vi "Teleop.vi"(10 "Match Info":T1={"Autonomous Elapsed Seconds"=0.0, "TeleOp Elapsed Seconds"=0.0, "Disabled Elapsed Seconds"=0.0, "Visited Autonomous"=FALSE, "Visited TeleOp"=FALSE, "Visited Disabled"=FALSE, "Autonomous Settings"={"Autonomous Style"=enum."Independent", "VI Refnum"=refnum}}, 11 "Call Context":T2) -> ()   [LabVIEW 2016]
doc: "This VI is called for each TeleOp packet received from the DS where the robot is not disabled. It is often used to read from the joysticks and update I/O or to update setpoints for timed control loops. It should complete and return within 20 milliseconds or it may miss DS packets."
uses:
  <vilib>/Rock Robotics/WPI/DriverStation/WPI_DriverStationDerivedRobotMode.ctl
  <vilib>/Rock Robotics/WPI/DriverStation/WPI_DriverStationMatch Info.ctl
  <vilib>/Rock Robotics/WPI/Solenoid/WPI_SolenoidValue.ctl
  <vilib>/Rock Robotics/WPI/Relay/WPI_RelayValue.ctl
  <vilib>/Rock Robotics/Network Tables/NT Read Boolean.vi
  <vilib>/Rock Robotics/Network Tables/NT Read Number.vi
  <vilib>/Rock Robotics/WPI/Utilities/WPI_GetSetVariantRefNum.vi
  <vilib>/Rock Robotics/Network Tables/NT Write Boolean Array.vi
  <vilib>/Rock Robotics/Network Tables/NT Write Numeric Array.vi
  <vilib>/Rock Robotics/WPI/RobotDrive/WPI_RobotDriveMecanumDrive_Cartesian.vi
  <vilib>/Rock Robotics/Network Tables/NT Write Boolean.vi
  <vilib>/Rock Robotics/WPI/Solenoid/WPI_SolenoidSetEnum.vi
  <vilib>/Rock Robotics/Network Tables/NT Write Number.vi
panel:
  out "Sample Slider 0":dbl(slide) scale=0.0..5.0
  out "Sample Boolean 1":bool
  out "Sample Boolean 0":bool
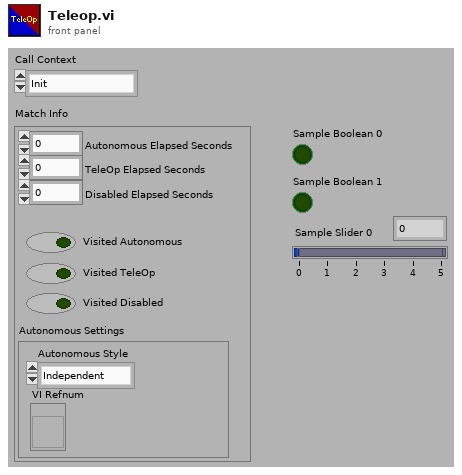
[diagram p1: front panel]
types:
  T1 = typedef "WPI_DriverStationMatch Info.ctl" = cluster{"Autonomous Elapsed Seconds":dbl, "TeleOp Elapsed Seconds":dbl, "Disabled Elapsed Seconds":dbl, "Visited Autonomous":bool, "Visited TeleOp":bool, "Visited Disabled":bool, "Autonomous Settings":cluster{"Autonomous Style":enum16{"Iterative", "Independent"}, "VI Refnum":refnum<vi>}}
  T2 = typedef "WPI_DriverStationDerivedRobotMode.ctl" = enum16{"Init", "Execute", "Stop"}
  T3 = typedef "WPI_SolenoidValue.ctl" = enum16{"Off", "On", "Forward", "Reverse"}
  T4 = typedef "WPI_MotorControlDeviceRef.ctl" = cluster{"DeviceStatus":errorcluster, "Type":T5, "PWM":cluster{"PWM Channel":T6, "DeadBand":T7}, "CAN":cluster{"Device Number":u8, "SetOutput VI Ref":variant, "GetOutput VI Ref":variant, "Enable VI Ref":variant, "Disable VI Ref":variant, "Data":variant}, "Invert":bool}
  T5 = typedef "WPI_MotorControlType.ctl" = enum16{"PWM", "CAN"}
  T6 = typedef "FPGA_DIOPWMChannel.ctl" = enum8{"PWM 0", "PWM 1", "PWM 2", "PWM 3", "PWM 4", "PWM 5", "PWM 6", "PWM 7", "PWM 8", "PWM 9", "PWM MXP 0", "PWM MXP 1", "PWM MXP 2", "PWM MXP 3", "PWM MXP 4", "PWM MXP 5", "PWM MXP 6", "PWM MXP 7", "PWM MXP 8", "PWM MXP 9", "Invalid"}
  T7 = typedef "WPI_PWMDeadband.ctl" = cluster{"Name":string, "maxPositivePwm":i32, "minPositivePwm":i32, "centerPwm":i32, "maxNegativePwm":i32, "minNegativePwm":i32, "angularRange":u16}
  T8 = typedef "WPI_JoystickDevRef.ctl" = cluster{"Device":T9}
  T9 = typedef "WPI_JoystickDeviceEnum.ctl" = enum16{"USB 0", "USB 1", "USB 2", "USB 3", "USB 4", "USB 5"}
  T10 = typedef "WPI_SolenoidDevRef.ctl" = cluster{"DevStatus":errorcluster, "Pneumatics Control Module":u8, "Forward Solenoid Channel":T11, "Reverse Solenoid Channel":T11}
  T11 = typedef "WPI_SolenoidChannel.ctl" = enum8{"Solenoid 0", "Solenoid 1", "Solenoid 2", "Solenoid 3", "Solenoid 4", "Solenoid 5", "Solenoid 6", "Solenoid 7", "Invalid"}
  T12 = typedef "WPI_RobotDriveDevRef.ctl" = cluster{"DevStatus":errorcluster, "Motors[]":T4[], "Square Inputs":bool, "Max Output":dbl}
  T13 = typedef "WPI_CompressorDevRef.ctl" = cluster{"DevStatus":errorcluster, "Pneumatics Control Module":u8}
  T14 = typedef "WPI_RelayValue.ctl" = enum16{"Off", "On", "Forward", "Reverse"}
  T15 = typedef "WPI_RelayDevRef.ctl" = cluster{"DevStatus":errorcluster, "Relay Channel":T16, "Relay Direction":T17}
  T16 = typedef "FPGA_DIORelayChannel.ctl" = enum8{"Relay 0", "Relay 1", "Relay 2", "Relay 3", "Invalid"}
  T17 = typedef "WPI_RelayDirection.ctl" = enum16{"Both directions", "Forward only", "Reverse only"}
  T18 = cluster{"Yaw":dbl, "Roll":dbl, "Pitch":dbl, "Heading":dbl, "Fused Heading":dbl}
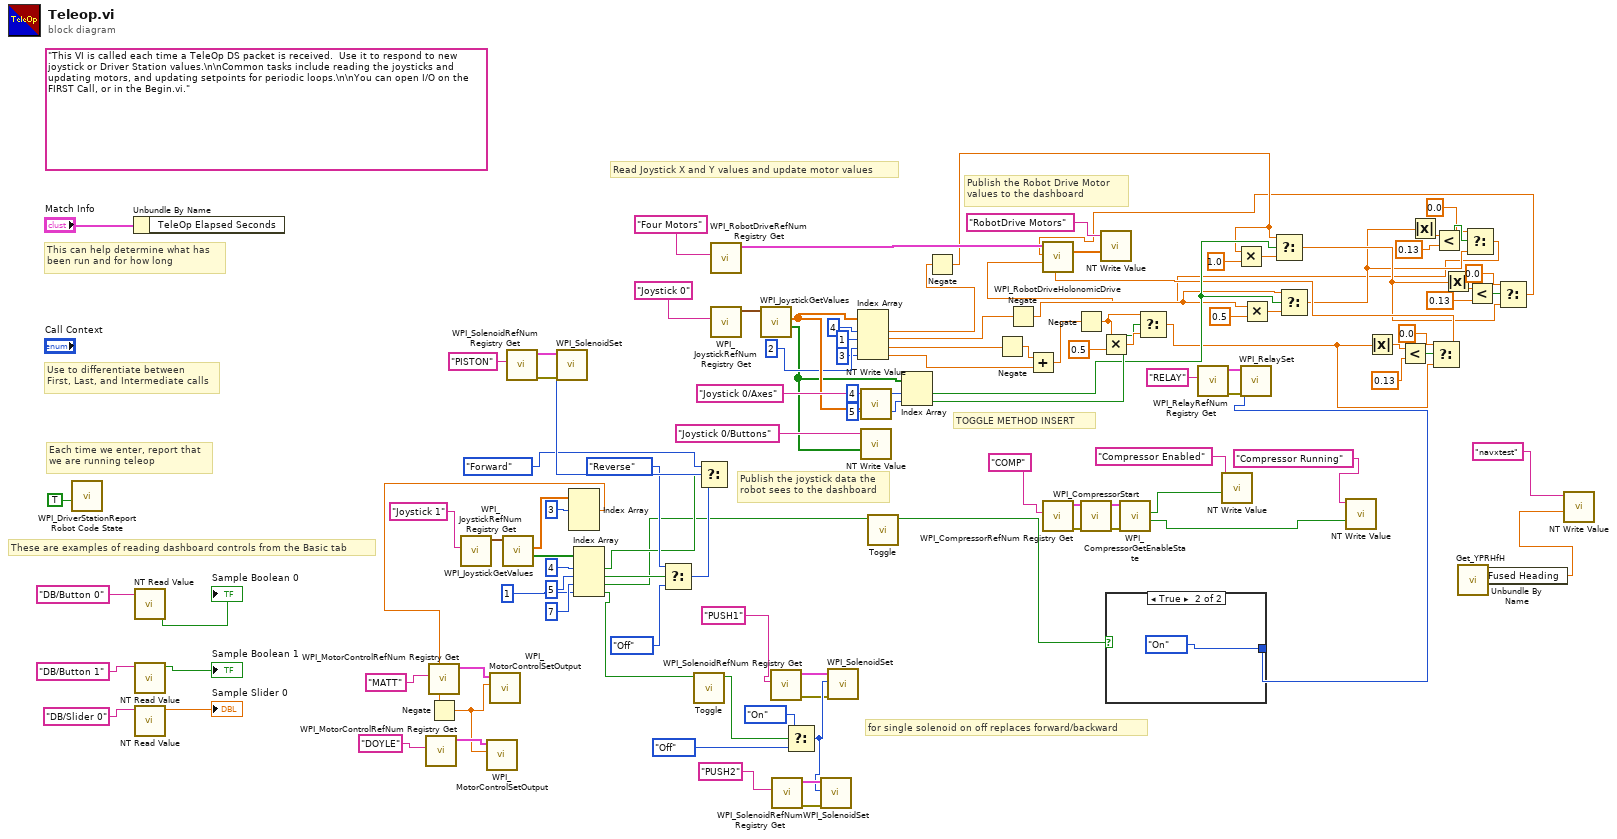
[diagram p0: block diagram]
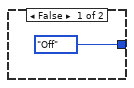
[diagram p2: hidden frame]
diagram:
  (unwired) "This VI is called each time a TeleOp DS packet is received.  Use it to respond to new joystick or Driver Station values.\n\nCommon tasks include reading the joysticks and updating motors, and updating setpoints for periodic loops.\n\nYou can open I/O on the FIRST Call, or in the Begin.vi."
  # "for single solenoid on off replaces forward/backward"
  # "TOGGLE METHOD INSERT"
  # "Publish the Robot Drive Motor\nvalues to the dashboard"
  # "Publish the joystick data the\nrobot sees to the dashboard"
  # "Read Joystick X and Y values and update motor values"
  # "These are examples of reading dashboard controls from the Basic tab"
  # "Each time we enter, report that\nwe are running teleop"
  # "Use to differentiate between\nFirst, Last, and Intermediate calls"
  # "This can help determine what has\nbeen run and for how long"
  n1 = call <vilib>:"WPI_DriverStationReport Robot Code State.vi"("TeleOp"=TRUE ("Autonomous")) -> ()  [unwired: 10 in, 1 out]
  n2 = Unbundle By Name("Match Info") -> ()  [unwired: 1 out]
  n3 = call-poly <vilib>:"NT Read Value.vi"("Name"="DB/Button 0" ("refnum name")) -> ("Boolean"=→"Sample Boolean 0":bool)  [unwired: 9 in, 1 out]
  n4 = call-poly <vilib>:"NT Read Value.vi"("Name"="DB/Button 1" ("refnum name")) -> ("Boolean"=→"Sample Boolean 1":bool)  [unwired: 9 in, 1 out]
  n5 = call-poly <vilib>:"NT Read Value.vi"("Name"="DB/Slider 0" ("refnum name")) -> ("Numeric"=→"Sample Slider 0":dbl)  [unwired: 9 in, 1 out]
  n6 = call <vilib>:"WPI_MotorControlRefNum Registry Get.vi"("refnum name"="DOYLE") -> ("MotorControlDevRef"=w15:T4)  [unwired: 9 in, 1 out]
  n7 = call <vilib>:"WPI_MotorControlRefNum Registry Get.vi"("refnum name"="MATT") -> ("MotorControlDevRef"=w14:T4)  [unwired: 9 in, 1 out]
  n8 = call <vilib>:"WPI_JoystickRefNum Registry Get.vi"("refnum name"="Joystick 1") -> ("JoystickDevRef"=w85:T8)  [unwired: 1 in, 9 out]
  n9 = call <vilib>:"WPI_JoystickGetValues.vi"("JoystickDevRef"=w85) -> ("Buttons"=w84:bool[], "Axes"=w71:dbl[])  [unwired: 6 in, 3 out]
  n10 = call <vilib>:"WPI_SolenoidRefNum Registry Get.vi"("refnum name"="PISTON") -> ("error out"=w80:errorcluster, "SolenoidDevRef"=w79:T10)  [unwired: 9 in]
  n11 = Index Array(array=w71, index #1=3 ("index")) -> (element #1=w69:dbl)  [unwired: 2 in, 2 out]
  n12 = Negate(x=w69) -> (-x=w13:dbl)
  n13 = call <vilib>:"WPI_MotorControlSetOutput.vi"("Output"=w13, "MotorControlDevRef"=w15) -> ()  [unwired: 7 in, 3 out]
  n14 = call <vilib>:"WPI_MotorControlSetOutput.vi"("Output"=w13, "MotorControlDevRef"=w14) -> ()  [unwired: 7 in, 3 out]
  n15 = Index Array(array=w84, index #1=4 ("index"), index #2=5 ("index"), index #3=7 ("index"), index #4=1 ("index")) -> (element #1=w73:bool, element #2=w72:bool, element #3=w67:bool, element #4=w7:bool)
  n16 = Select(t=WPI_SolenoidValue."Reverse" ("Value"), s=w72, f=WPI_SolenoidValue."Off" ("Value")) -> (s? t:f=w76:T3)
  n17 = call "Toggle.vi"("Button Input"=w7) -> ("Toggle Output"=w6:bool)  [unwired: 9 in, 1 out]
  n18 = Select(t=WPI_SolenoidValue."Forward" ("Value"), s=w73, f=w76) -> (s? t:f=w78:T3)
  n19 = call-poly <vilib>:"WPI_SolenoidSet.vi"("error in (no error)"=w80, "Value"=w78, "SolenoidDevRef"=w79) -> ()  [unwired: 7 in, 2 out]
  n20 = call <vilib>:"WPI_RobotDriveRefNum Registry Get.vi"("refnum name"="Four Motors") -> ("RobotDriveDevRef"=w104:T12)  [unwired: 1 in, 9 out]
  n21 = call <vilib>:"WPI_JoystickRefNum Registry Get.vi"("refnum name"="Joystick 0") -> ("JoystickDevRef"=w102:T8)  [unwired: 1 in, 9 out]
  n22 = call <vilib>:"WPI_JoystickGetValues.vi"("JoystickDevRef"=w102) -> ("Buttons"=w57:bool[], "Axes"=w100:dbl[])  [unwired: 6 in, 3 out]
  n23 = call <vilib>:"WPI_SolenoidRefNum Registry Get.vi"("refnum name"="PUSH1") -> ("error out"=w1:errorcluster, "SolenoidDevRef"=w9:T10)  [unwired: 9 in]
  n24 = call <vilib>:"WPI_SolenoidRefNum Registry Get.vi"("refnum name"="PUSH2") -> ("error out"=w2:errorcluster, "SolenoidDevRef"=w10:T10)  [unwired: 9 in]
  n25 = Select(t=WPI_SolenoidValue."On" ("Value"), s=w6, f=WPI_SolenoidValue."Off") -> (s? t:f=w4:T3)
  n26 = call-poly <vilib>:"WPI_SolenoidSet.vi"("error in (no error)"=w2, "Value"=w4, "SolenoidDevRef"=w10) -> ()  [unwired: 7 in, 2 out]
  n27 = call-poly <vilib>:"WPI_SolenoidSet.vi"("error in (no error)"=w1, "Value"=w4, "SolenoidDevRef"=w9) -> ()  [unwired: 7 in, 2 out]
  n28 = Index Array(array=w100, index #1=4 ("index"), index #2=1 ("index"), index #3=2 ("index"), index #4=3 ("index")) -> (element #1=w95:dbl, element #2=w96:dbl, element #3=w90:dbl, element #4=w88:dbl)
  n29 = call-poly <vilib>:"NT Write Value.vi"("Numeric Array"=w100, "Name"="Joystick 0/Axes") -> ()  [unwired: 9 in, 1 out]
  n30 = call-poly <vilib>:"NT Write Value.vi"("Boolean Array"=w57, "Name"="Joystick 0/Buttons") -> ()  [unwired: 9 in, 1 out]
  n31 = call "Toggle.vi"("Button Input"=w67) -> ("Toggle Output"=w62:bool)  [unwired: 9 in, 1 out]
  n32 = Index Array(array=w57, index #1=4 ("index"), index #2=5 ("index")) -> (element #1=w48:bool, element #2=w49:bool)
  n33 = Negate(x=w95) -> (-x=w47:dbl)
  n34 = Negate(x=w90) -> (-x=w89:dbl)
  n35 = Negate(x=w96) -> (-x=w44:dbl)
  n36 = Add(x=w89, y=w88) -> (x+y=w87:dbl)
  n37 = call <vilib>:"WPI_CompressorRefNum Registry Get.vi"("refnum name"="COMP") -> ("error out"=w21:errorcluster, "CompressorDevRef"=w20:T13)  [unwired: 9 in]
  n38 = Negate(x=w87) -> (-x=w52:dbl)
  n39 = call <vilib>:"WPI_CompressorStart.vi"("error in (no error)"=w21, "CompressorDevRef"=w20) -> ("error out"=w19:errorcluster, "CompressorDevRef"=w18:T13)  [unwired: 8 in]
  n40 = Multiply(x=w52, y=0.5) -> (x*y=w53:dbl)
  n41 = case shown="True" w62 {
    tunnel: [WPI_RelayValue."Off" ("RelayValue") WPI_RelayValue."On" ("RelayValue")] -> w58
    frame False {
    }
    frame True {
    }
  }
  n42 = call <vilib>:"WPI_CompressorGetEnableState.vi"("error in (no error)"=w19, "CompressorDevRef"=w18) -> ("Compressor Running"=w63:bool, "Enabled"=w64:bool)  [unwired: 6 in, 2 out]
  n43 = Select(t=w52, s=w49, f=w53) -> (s? t:f=w31:dbl)
  n44 = call <vilib>:"WPI_RelayRefNum Registry Get.vi"("refnum name"="RELAY") -> ("error out"=w60:errorcluster, "RelayDevRef"=w59:T15)  [unwired: 9 in]
  n45 = call-poly <vilib>:"NT Write Value.vi"("Boolean"=w64, "Name"="Compressor Enabled") -> ()  [unwired: 9 in, 1 out]
  n46 = Multiply(x=w47, y=1.0) -> (x*y=w54:dbl)
  n47 = call <vilib>:"WPI_RelaySet.vi"("error in (no error)"=w60, "RelayValue"=w58, "RelayDevRef"=w59) -> ()  [unwired: 7 in, 2 out]
  n48 = Multiply(x=w44, y=0.5) -> (x*y=w50:dbl)
  n49 = Select(t=w47, s=w48, f=w54) -> (s? t:f=w29:dbl)
  n50 = Select(t=w44, s=w48, f=w50) -> (s? t:f=w27:dbl)
  n51 = call-poly <vilib>:"NT Write Value.vi"("Boolean"=w63, "Name"="Compressor Running") -> ()  [unwired: 9 in, 1 out]
  n52 = Absolute Value(x=w31) -> (abs(x)=w40:dbl)
  n53 = Less?(x=w40, y=0.13) -> (x < y?=w43:bool)
  n54 = Absolute Value(x=w27) -> (abs(x)=w36:dbl)
  n55 = Select(t=0.0, s=w43, f=w31) -> (s? t:f=w30:dbl)
  n56 = Less?(x=w36, y=0.13) -> (x < y?=w41:bool)
  n57 = Absolute Value(x=w29) -> (abs(x)=w35:dbl)
  n58 = call <vilib>:"Get_YPRHfH.vi"() -> ("YRPHfH"=w24:T18)  [unwired: 11 in]
  n59 = Select(t=0.0, s=w41, f=w27) -> (s? t:f=w26:dbl)
  n60 = Unbundle By Name(w24) -> ("Fused Heading"=w23:dbl)
  n61 = Less?(x=w35, y=0.13) -> (x < y?=w42:bool)
  n62 = Select(t=0.0, s=w42, f=w29) -> (s? t:f=w28:dbl)
  n63 = call-poly <vilib>:"WPI_RobotDriveHolonomicDrive.vi"("Rotation"=w30, "Y"=w26, "X"=w28, "RobotDriveDevRef"=w104) -> ("Motor Values"=w98:dbl[])  [unwired: 5 in, 2 out]
  n64 = call-poly <vilib>:"NT Write Value.vi"("Numeric Array"=w98, "Name"="RobotDrive Motors") -> ()  [unwired: 9 in, 1 out]
  n65 = call-poly <vilib>:"NT Write Value.vi"("Numeric"=w23, "Name"="navxtest") -> ()  [unwired: 9 in, 1 out]
